vi "chat completions image (OpenAI).vi"(6 "timeout (600000)":i32=600000, 8 "error in":errorcluster, 9 "chat-completion req":T1={"model"="", "messages"=[], "max_tokens"=4096, "temperature"=0.8, "stream"=FALSE}, 10 "API url":string, 11 "Refnum in":T5) -> (0 "error out":errorcluster, 2 "Answer content":string, 3 "Refnum out":T5, 4 "reasoning content":string)   [LabVIEW 2023, in "LabVIEW LLM.lvlib"]
uses:
  LabVIEW LLM.lvlib
  <vilib>/httpClient/ClientHandle.ctl
  chat-completion complex req.ctl
  openai_complex_message.ctl
  chat-role.ctl
  complex content.ctl
  <vilib>/httpClient/POSTBuffer.vi
  <vilib>/httpClient/LabVIEWHTTPClient.lvlib
  <vilib>/addons/_JKI.lib/Serialization/JSON/JKI JSON Serialization.lvlib
  labview-ai-share/LabVIEW AI Base.lvlib
panel:
  out "Request JSON":string
  out "Response JSON":string
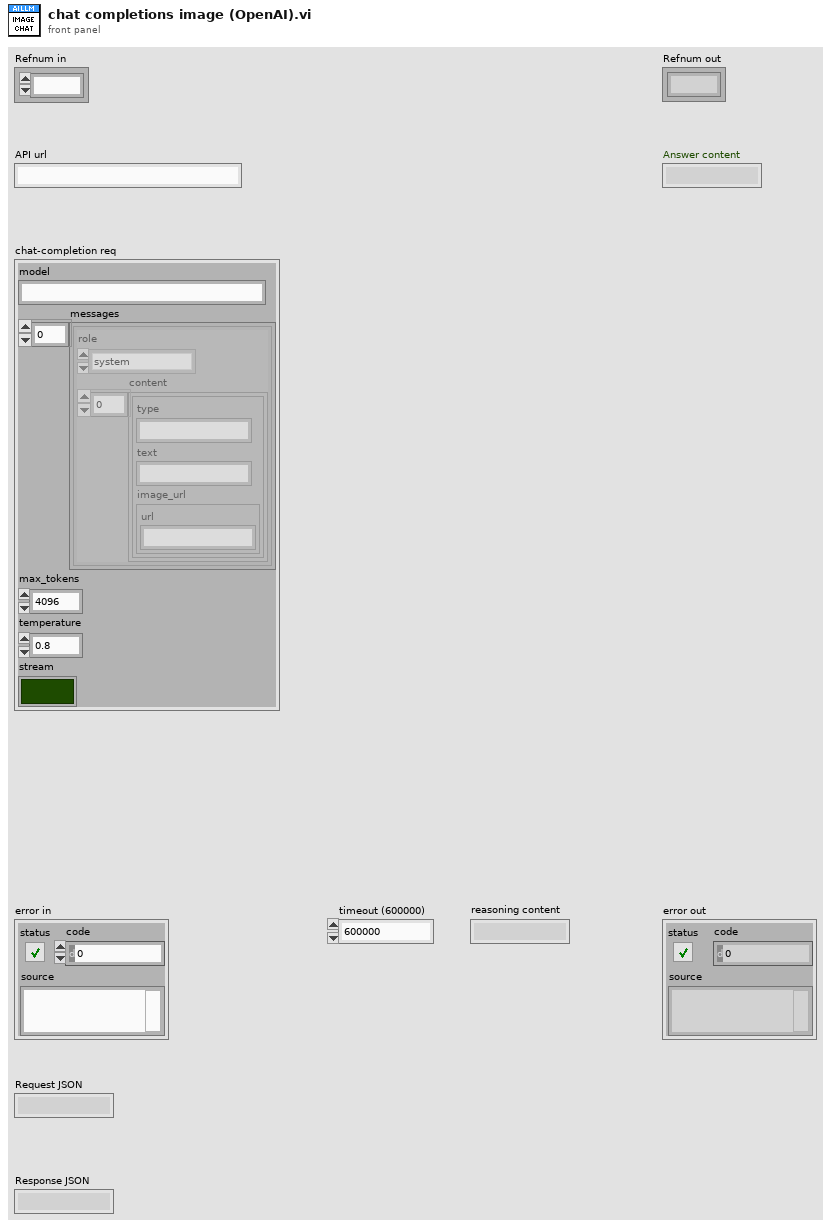
[diagram p1: front panel]
types:
  T1 = typedef "LabVIEW LLM.lvlib/chat-completion complex req.ctl" = cluster{"model":string, "messages":T2[], "max_tokens":u32, "temperature":dbl, "stream":bool}
  T2 = typedef "LabVIEW LLM.lvlib/openai_complex_message.ctl" = cluster{"role":T3, "content":T4[]}
  T3 = typedef "LabVIEW LLM.lvlib/chat-role.ctl" = enum16{"system", "user", "assistant"}
  T4 = typedef "LabVIEW LLM.lvlib/complex content.ctl" = cluster{"type":string, "text":string, "image_url":cluster{"url":string}}
  T5 = typedef "LabVIEWHTTPClient.lvlib/ClientHandle.ctl" = refnum<k1>
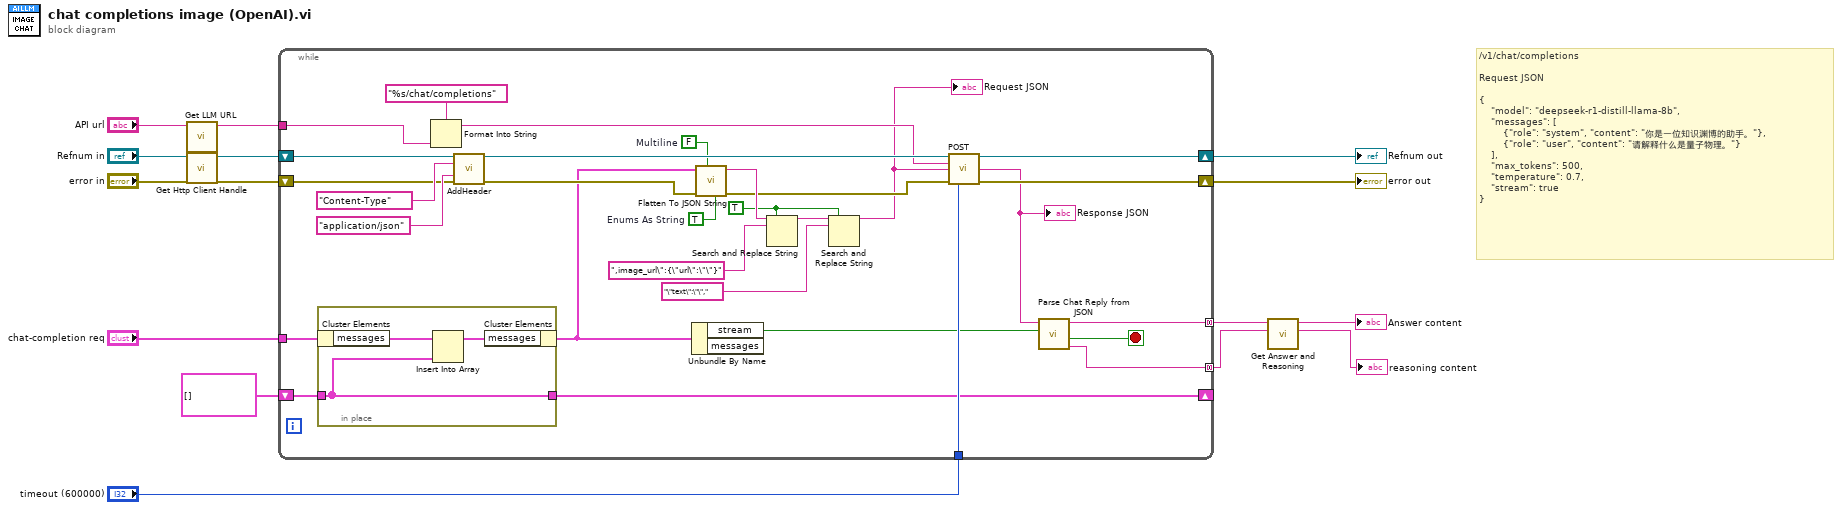
[diagram p0: block diagram]
diagram:
  # "/v1/chat/completions\n\nRequest JSON\n\n{\n    \"model\": \"deepseek-r1-distill-llama-8b\",\n    \"messages\": [\n        {\"role\": \"system\", \"content\": \"你是一位知识渊博的助手。\"},\n        {\"role\": \"user\", \"content\": \"请解释什么是量子物理。\"}\n    ],\n    \"max_tokens\": 500,\n    \"temperature\": 0.7,\n    \"stream\": true\n}"
  n1 = call "Get LLM URL.vi"("OpenAI API URL"="API url") -> ("OpenAI API URL"=w5:string)  [unwired: 10 in]
  n2 = call "Get Http Client Handle.vi"("Refnum in"="Refnum in") -> ("Refnum out"=w4:T5)  [unwired: 10 in]
  n3 = while {
    tunnel: "timeout (600000)" -> [w44]
    tunnel: "chat-completion req" -> [w35]
    tunnel: w5 -> [w32]
    shift-right: [w36] -> w11
    shift-left: w4 -> [w38]
    shift-right: [w43] -> w13
    shift-left: "error in" -> [w33]
    tunnel: [w25] -> w7 mode=concatenating
    shift-right: [w21] -> _
    shift-left: T2[] [] ("Array") -> [w24]
    tunnel: [w20] -> w3 mode=concatenating
    stop <- w26 stop-if-true
    w15 = TRUE ("replace all? (F)")
    w28 = TRUE  # Enums As String
    w29 = FALSE  # Multiline
    n4 = in-place {
      in-place-border: w24 -> [w45]
      in-place-border: [w45] -> w21
      n5 = in-place-cluster #1(w35) -> ("messages"=w47:T2[])
      n6 = Insert Into Array(array=w47, new element=w45) -> (w46:T2[])  [unwired: 1 in]
      n7 = in-place-cluster #1("messages"=w46) -> (w23:T1)
    }
    n8 = Format Into String(format string="%s/chat/completions" ("url"), w32) -> (resulting string=w30:string)  [unwired: 2 in, 1 out]
    n9 = call <vilib>:"AddHeader.vi"("client handle"=w38, "header"="Content-Type", "value"="application/json", "error in (no error)"=w33) -> ("client handle out"=w39:T5, "error out"=w37:errorcluster)  [unwired: 10 in]
    n10 = Unbundle By Name(w23) -> ("stream"=w22:bool)  [unwired: 1 out]
    n11 = call <vilib>:"Flatten To JSON String.vi"("Enums As String (F)"=w28, "Multiline (T)"=w29, "error in"=w37, "Variant"=w23) -> ("error out"=w34:errorcluster, "JSON String"=w42:string)  [unwired: 6 in]
    n12 = Search and Replace String(replace all?=w15, input string=w42, search string=",image_url\":{\"url\":\"\"}") -> (result string=w19:string)  [unwired: 5 in, 3 out]
    n13 = Search and Replace String(replace all?=w15, input string=w19, search string="\"text\":\"\",") -> (result string=w18:string)  [unwired: 5 in, 3 out]
    "Request JSON" <- w18
    n14 = call-poly <vilib>:"POST.vi"("client handle"=w39, "url"=w30, "buffer"=w18, "error in (no error)"=w34, "timeout (10000)"=w44) -> ("client handle out"=w36:T5, "body"=w27:string, "error out"=w43:errorcluster)  [unwired: 7 in, 1 out]
    "Response JSON" <- w27
    n15 = call "Parse Chat Reply from JSON.vi"("stream"=w22, "Response JSON"=w27) -> ("openrouter reasoning"=w20:string, "complete?"=w26:bool, "answer"=w25:string)  [unwired: 6 in, 1 out]
  }
  "error out" <- w13
  "Refnum out" <- w11
  n16 = call "Get Answer and Reasoning.vi"("openrouter reasoning"=w3, "answer"=w7) -> ("reasoning"=→"reasoning content":string, "answer"=→"Answer content":string)  [unwired: 8 in]
